vi "Text Get Sections.vi"(8 "Error In":errorcluster, 11 "Receipt Lines":string[](array[string])) -> (0 "Error Out":errorcluster, 1 "Footer":string[](array[string]), 2 "Main Body":string[](array[string]), 3 "Header":string[](array[string]), 5 "Line Numbers":T1)   [LabVIEW 2018, in "Receipt Parsing.lvlib"]
uses:
  Receipt Parsing.lvlib
  Line Number.ctl
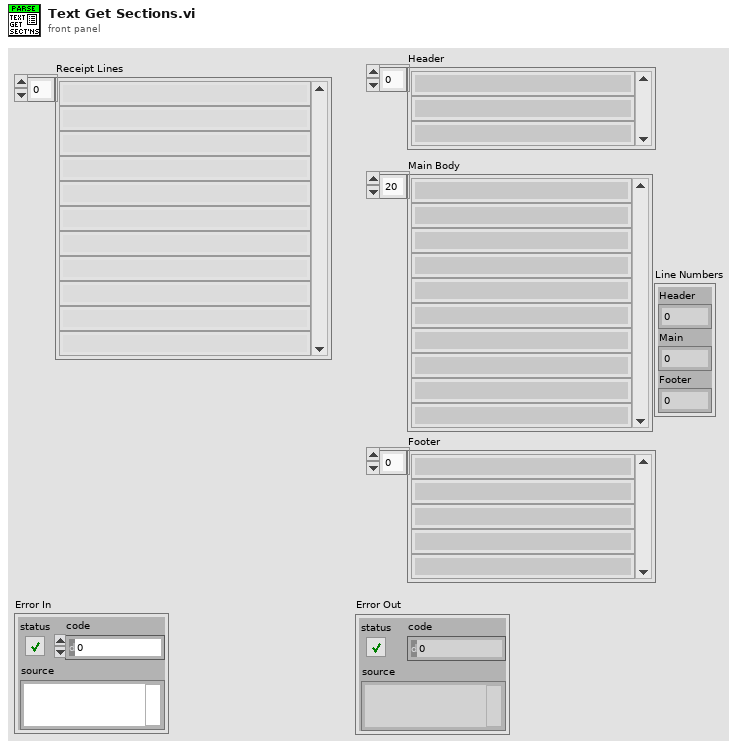
[diagram p1: front panel]
types:
  T1 = typedef "Receipt Parsing.lvlib/Line Number.ctl" = cluster{"Header":i32, "Main":i32, "Footer":i32}
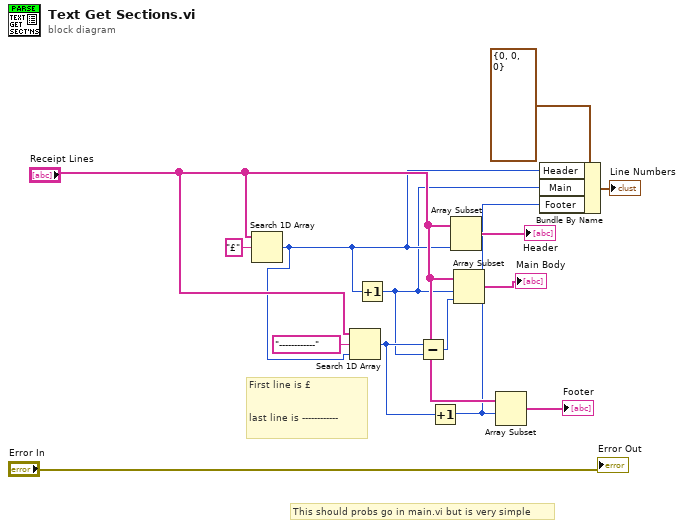
[diagram p0: block diagram]
diagram:
  # "This should probs go in main.vi but is very simple"
  # "First line is £\n\n\nlast line is ------------"
  n1 = Search 1D Array(1D array="Receipt Lines", element="£") -> (index of element=w4:i32)  [unwired: 1 in]
  n2 = Search 1D Array(1D array="Receipt Lines", element="------------", start index (0)=w4) -> (index of element=w6:i32)
  n3 = Increment(x=w4) -> (x+1=w3:i32)
  n4 = Subtract(x=w6, y=w3) -> (x-y=w8:i32)
  n5 = Increment(x=w6) -> (x+1=w2:i32)
  n6 = Array Subset(array="Receipt Lines", length=w4) -> (→"Header":string[])  [unwired: 1 in]
  n7 = Array Subset(array="Receipt Lines", index=w3, length=w8) -> (→"Main Body":string[])
  n8 = Array Subset(array="Receipt Lines", index=w2) -> (→"Footer":string[])  [unwired: 1 in]
  n9 = Bundle By Name(cluster=T1 {"Header"=0, "Main"=0, "Footer"=0} ("Line Number"), "Header"=w4, "Main"=w3, "Footer"=w2) -> (→"Line Numbers":T1)
  "Error Out" <- "Error In"
